vi "Construct Build VIPB Step.vi"(5 "Build VIPB Step in":refnum<class "Build VIPB Step.lvclass">, 8 "error in (no error)":errorcluster, 11 "Path":path) -> (0 "error out":errorcluster, 3 "Build VIPB Step":refnum<class "Build VIPB Step.lvclass">)   [LabVIEW 2019, in "VIPM.lvlib" / "Build VIPB Step.lvclass"]
uses:
  Build VIPB Step.lvclass
  Build VIPB Step.lvclass/Build VIPB Step.ctl
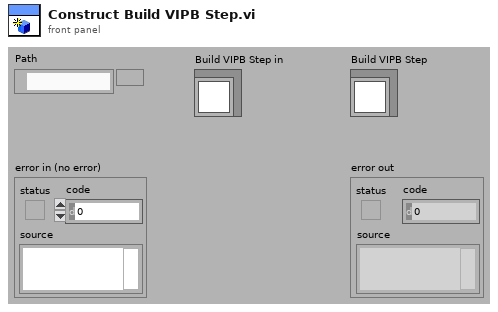
[diagram p1: front panel]
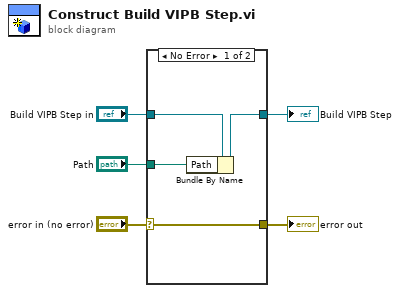
[diagram p0: block diagram]
diagram:
  n1 = case shown="No Error" "error in (no error)" {
    selector: "error in (no error)" -> [w9 w11]
    tunnel: [w9 w11] -> w4
    tunnel: [w7 w10] -> w2
    tunnel: "Build VIPB Step in" -> [w8 w10]
    tunnel: "Path" -> [w6 _]
    frame No Error {
      n2 = Bundle By Name(cluster=w8, "Path"=w6) -> (w7:refnum<class "Build VIPB Step.lvclass">)
    }
    frame Error {
    }
  }
  "error out" <- w4
  "Build VIPB Step" <- w2
